vi "single use states FG.vi"(6 "exit in":bool, 8 "state # in":i32, 10 "substate":T1, 11 "menu (get)":enum16{"set", "get"}(ring)=enum."get") -> (0 "first call?":bool, 1 "exit out":bool, 2 "state # out":i32, 3 "substate out":T1)   [LabVIEW 2013]
uses:
  typedefs/singleUseSubstate.ctl
panel:
  # "The All-Powerful Functional Global with all the States (Single Use)"
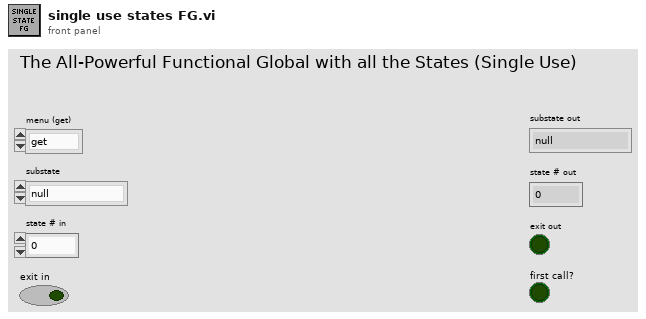
[diagram p1: front panel]
types:
  T1 = typedef "singleUseSubstate.ctl" = enum16{"null", "wait", "shift high", "shift low", "extend shooter", "retract shooter", "latch", "unlatch", "end"}
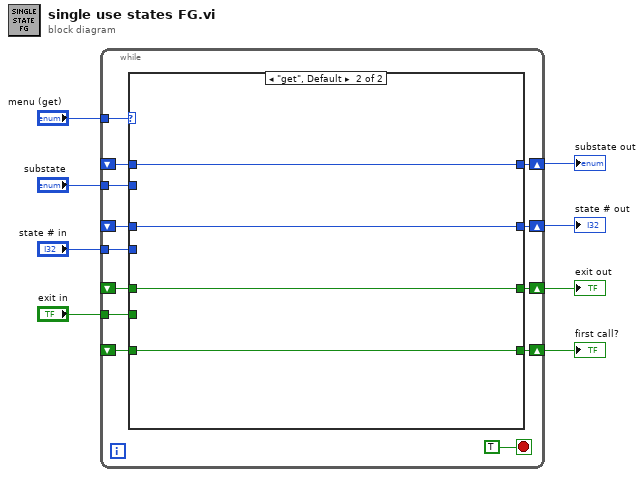
[diagram p0: block diagram]
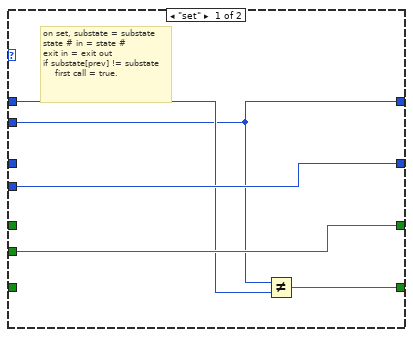
[diagram p2: hidden frame]
diagram:
  n1 = while {
    tunnel: "menu (get)" -> [w21]
    shift-right: [w17] -> w4
    shift-left: _ -> [w18]
    shift-right: [w16] -> w3
    shift-left: _ -> [w19]
    tunnel: "substate" -> [w15]
    tunnel: "state # in" -> [w14]
    shift-right: [w13] -> w2
    shift-left: _ -> [w12]
    tunnel: "exit in" -> [w11]
    shift-right: [w10] -> w1
    shift-left: _ -> [w9]
    stop <- TRUE stop-if-true
    n2 = case shown="\"get\", Default" w21 {
      tunnel: w19 -> [_ w29]
      tunnel: w18 -> [w23 w30]
      tunnel: [w22 w30] -> w17
      tunnel: [w26 w29] -> w16
      tunnel: w15 -> [w22 _]
      tunnel: w14 -> [w26 _]
      tunnel: [w25 w28] -> w13
      tunnel: w12 -> [_ w28]
      tunnel: w11 -> [w25 _]
      tunnel: [w24 w27] -> w10
      tunnel: w9 -> [_ w27]
      frame "set" {
        # "on set, substate = substate\nstate # in = state #\nexit in = exit out\nif substate[prev] != substate\n    first call = true."
        n3 = Not Equal?(x=w22, y=w23) -> (x != y?=w24:bool)
      }
      frame "get", Default {
      }
    }
  }
  "state # out" <- w3
  "exit out" <- w2
  "first call?" <- w1
  "substate out" <- w4
